vi "ExtTrigAuger.vi"() -> ()   [LabVIEW 2014]
uses:
  FPGA state.ctl
  <vilib>/Platform/TimedLoop/XDataNode/timing_clust.ctl
  <vilib>/Platform/TimedLoop/XDataNode/nitl_modes.ctl
  <vilib>/Platform/TimedLoop/XDataNode/wakeup.ctl
  <vilib>/rvi/Emulation/niFpgaSctlEmulationGetInTimedLoop.vi
  <vilib>/rvi/Emulation/niFpgaEmulationReportErrorSimple.vi
  <vilib>/rvi/Emulation/niFpgaGetClockAttributes.vi
  <vilib>/rvi/Emulation/niFpgaCriticalErrorInLSC.vi
  <vilib>/rvi/eio/common/nirviEmuTemplateMethod_errors.vi
  <vilib>/rvi/interface/RandomDataEmulation/niFpgaRandomDataHandleErrors.vi
  <vilib>/Platform/TimedLoop/XDataNode/XDataNode.xnode
  <vilib>/eio/EIONode/EIONode.xnode
  <vilib>/rvi/DataTransferAndStorage/Container/XNode/niFpgaContainer.xnode
  <vilib>/rvi/interface/RandomDataEmulation/nirviRandomDataFpgaReadWriteTemplate.vi
  <vilib>/Platform/TimedLoop/XDataNode/XDNodeRunTimeDep.lvlib
panel:
  out "Overflow":bool
  in  "Trigger Mode":enum8{"Off", "PXI Trig0", "DIO-08 Trig"}(ring)
  # "Acquisition can be controlled by external trigger\n(through PXI backplane or input connector)\nor by the FPGA 25 MHz Clock."
  # "ExtTrig AugerCounter"
  # "Each U64 FIFO element is a pair of U32 with\n28 bits data, 4 bit ID in most significant bits\nID 0-7 for data channels, 8 for clock and 9 for trig count\n\nOn trigger return sample count, delta T in first element,\nand counts since last trigger on the eight data channels\n(7 for Auger plus aux) in the next 4 elements\n\nOn overflow, set trigger mode to off and flush FIFO\nOFF mode clears overflow, also resests sample count"
  # "Red for overflow\ngreen for normal"
  # "FPGA DMA-FIFO CANNOT be cleared by FPGA,\nonly by PC Host VI. Ctr Overflow will be on when\nFPGA-side FIFO is full!"
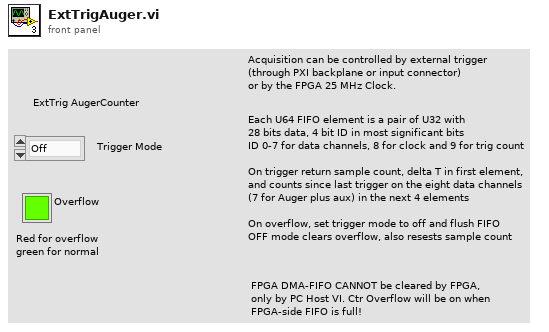
[diagram p1: front panel]
types:
  T1 = typedef "FPGA state.ctl" = enum8{"Wait", "Triggered", "Transfer 1", "Transfer 2", "Transfer 3", "Transfer 4", "Overflow"}
  T2 = typedef "XDNodeRunTimeDep.lvlib/timing_clust.ctl" = cluster{"Expected End [f-1]":u64, "Actual End [f-1]":u64, "Finished Late? [f-1]":bool, "Expected End [i-1]":u64, "Actual End [i-1]":u64, "Finished Late? [i-1]":bool, "Expected Start [i]":u64, "Actual Start [i]":u64, "Expected Start [f]":u64, "Actual Start [f]":u64, "Source Name":string, "Structure Name":string, "Period":i64, "Deadline":i64, "Offset":i64, "Start":i64, "Priority":i32, "Timeout":i32, "Mode":T3, "Wakeup Reason":T4, "Error":errorcluster, "Source Type":string, "Secondary Source Type":string, "Global End Time":u64, "Global Start Time":u64, "Frame Duration":u64, "Iteration Duration":u64, "Assigned CPU":i32, "I/O Scan Engine Mode":u32}
  T3 = typedef "XDNodeRunTimeDep.lvlib/nitl_modes.ctl" = enum32{"No Change", "Process missed periods, maintain original phase", "Discard missed periods, maintain original phase", "Process missed periods, ignore original phase", "Discard missed periods, ignore original phase"}
  T4 = typedef "XDNodeRunTimeDep.lvlib/wakeup.ctl" = enum32{"Normal", "Aborted", "Asynchronous wakeup", "Timing source error", "Timed loop error", "Timeout"}
  T5 = enum16{"Off", "PXI Trig0", "DIO-08 Trig", "Clocked"}
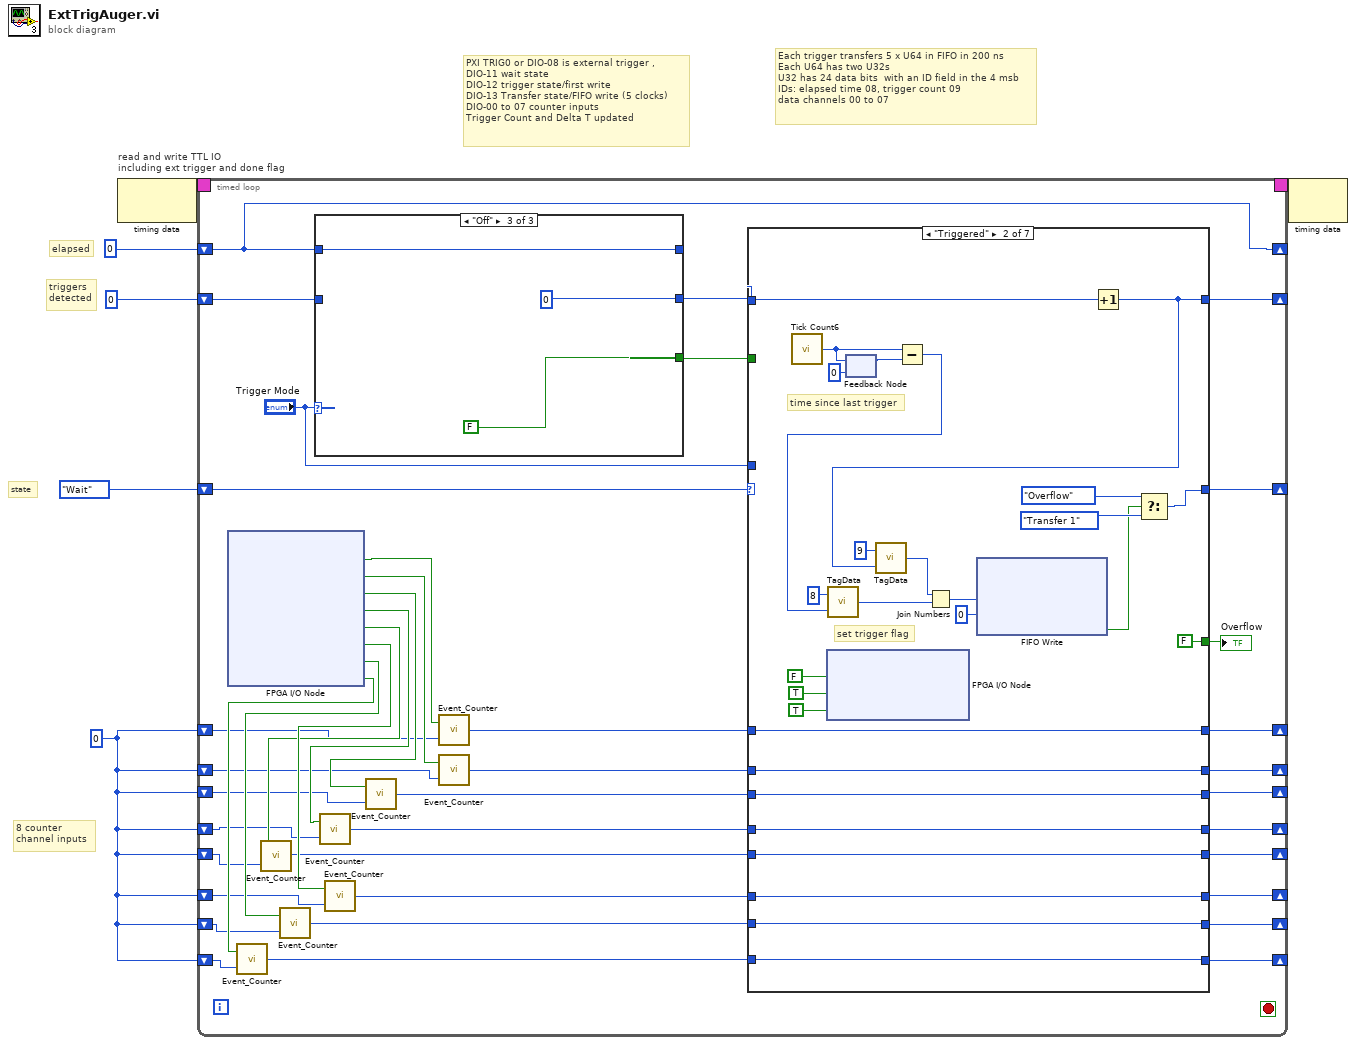
[diagram p0: block diagram]
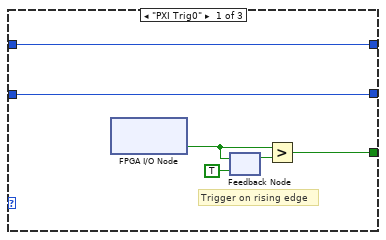
[diagram p2: hidden frame]
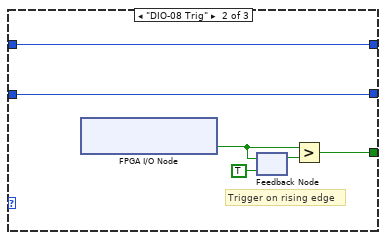
[diagram p3: hidden frame]
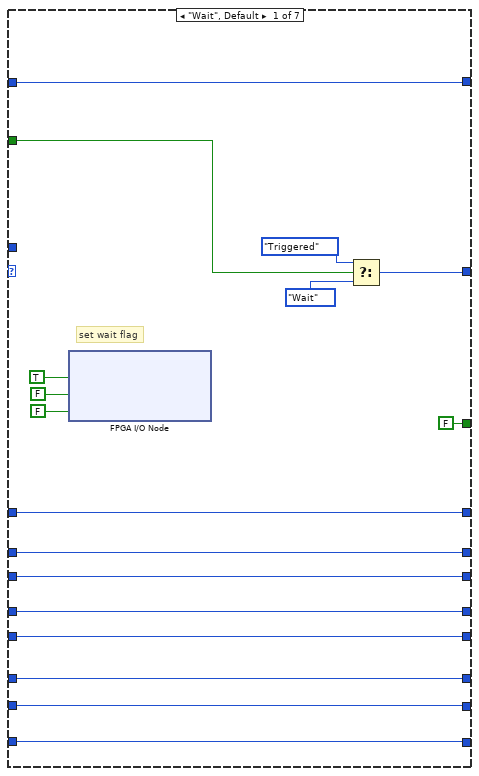
[diagram p4: hidden frame]
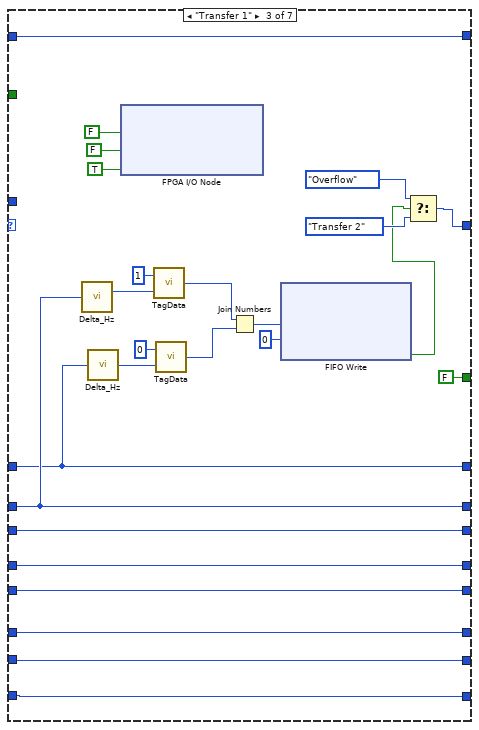
[diagram p5: hidden frame]
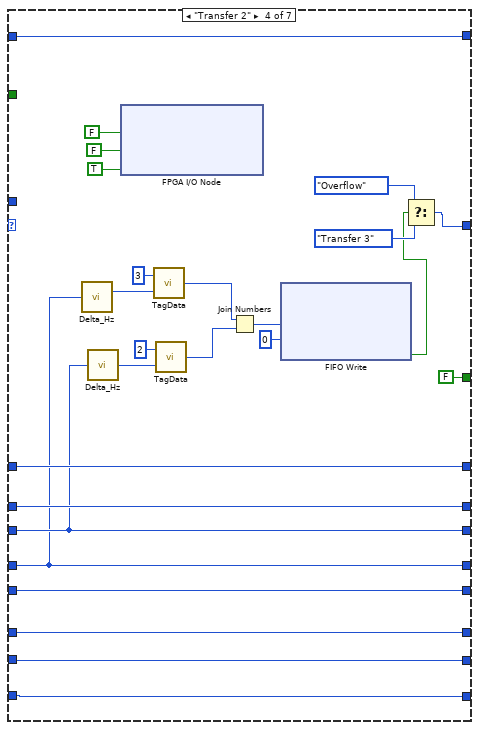
[diagram p6: hidden frame]
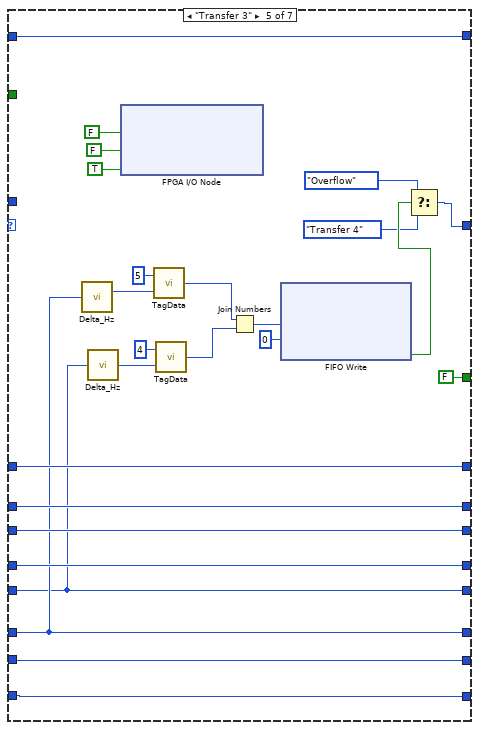
[diagram p7: hidden frame]
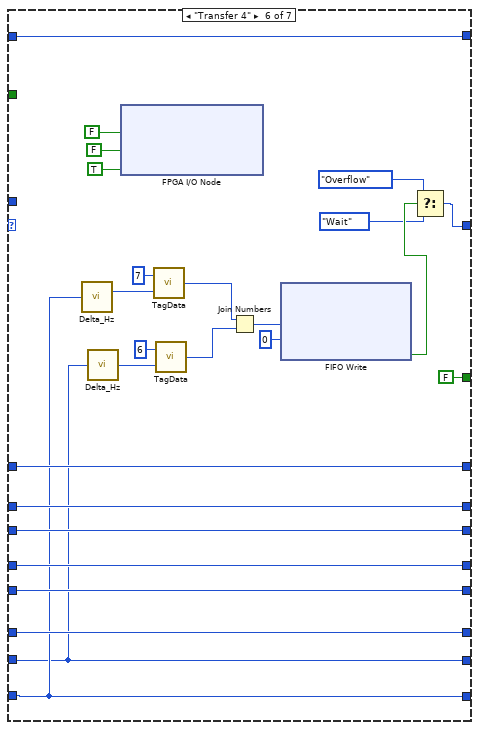
[diagram p8: hidden frame]
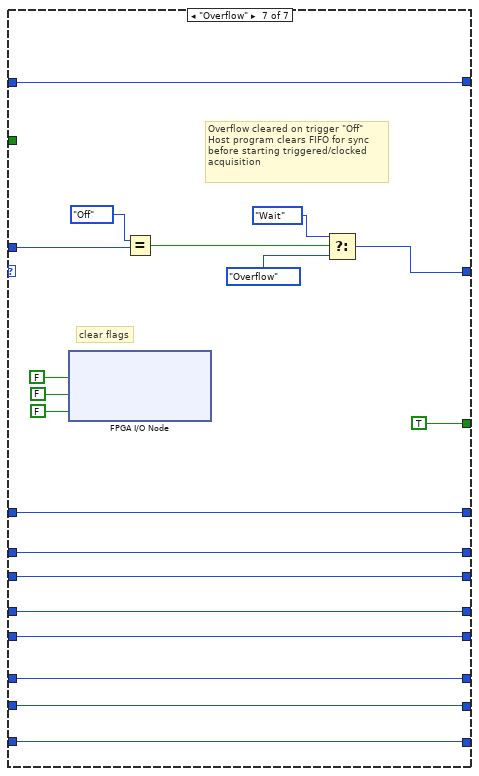
[diagram p9: hidden frame]
diagram:
  w1 = u32 0 ("Counts out")
  # "Each trigger transfers 5 x U64 in FIFO in 200 ns\nEach U64 has two U32s\nU32 has 24 data bits  with an ID field in the 4 msb\nIDs: elapsed time 08, trigger count 09\ndata channels 00 to 07"
  # "8 counter\nchannel inputs"
  # "elapsed"
  # "state"
  # "triggers\ndetected"
  # "PXI TRIG0 or DIO-08 is external trigger ,\nDIO-11 wait state\nDIO-12 trigger state/first write \nDIO-13 Transfer state/FIFO write (5 clocks)\nDIO-00 to 07 counter inputs \nTrigger Count and Delta T updated"
  n1 = node-c288() -> (w6:T2)  [unwired: 1 in]
  n2 = timed-loop "read and write TTL IO\nincluding ext trigger and done flag" {
    timing: w6 -> [_]
    timing-out: [_] -> w5
    shift-right: [w46] -> _
    shift-left: FPGA_state."Wait" -> [w47]
    shift-right: [w45] -> _
    shift-left: u32 0 -> [w11]
    shift-right: [w7] -> _
    shift-left: u32 0 -> [w7]
    shift-right: [w13] -> _
    shift-left: w1 -> [w29]
    shift-right: [w16] -> _
    shift-left: w1 -> [w30]
    shift-right: [w15] -> _
    shift-left: w1 -> [w34]
    shift-right: [w19] -> _
    shift-left: w1 -> [w35]
    shift-right: [w22] -> _
    shift-left: w1 -> [w38]
    shift-right: [w23] -> _
    shift-left: w1 -> [w37]
    shift-right: [w26] -> _
    shift-left: w1 -> [w39]
    shift-right: [w27] -> _
    shift-left: w1 -> [w40]
    stop <- _ stop-if-true
    n3 = xnode "FPGA I/O Node"() -> ("Connector0/DIO0"=w31:bool, "Connector0/DIO1"=w32:bool, "Connector0/DIO2"=w33:bool, "Connector0/DIO3"=w36:bool, "Connector0/DIO4"=w41:bool, "Connector0/DIO5"=w42:bool, "Connector0/DIO6"=w43:bool, "Connector0/DIO7"=w44:bool)  [unwired: 8 in, 8 out]
    n4 = call "Event_Counter.vi"("Counts in"=w40, "input"=w44) -> ("Counts out"=w28:u32)
    n5 = call "Event_Counter.vi"("Counts in"=w38, "input"=w41) -> ("Counts out"=w21:u32)
    n6 = call "Event_Counter.vi"("Counts in"=w39, "input"=w43) -> ("Counts out"=w25:u32)
    n7 = case shown="\"Off\"" "Trigger Mode" {
      tunnel: [w49 w56 FALSE ("Connector0/DIO8")] -> w8
      tunnel: w11 -> [w53 w59 _]
      tunnel: [w53 w59 u32 0] -> w9
      tunnel: w7 -> [w48 w54 w60]
      tunnel: [w48 w54 w60] -> _
      frame "PXI Trig0" {
        # "Trigger on rising edge"
        n8 = xnode "FPGA I/O Node"() -> ("TRIG0"=w50:bool)  [unwired: 1 in, 1 out]
        n9 = feedback #1(TRUE ("set")) -> (w51:bool)
        n10 = feedback-in #1(w50) -> ()
        n11 = Greater?(x=w50, y=w51) -> (0:w49:bool)
      }
      frame "DIO-08 Trig" {
        # "Trigger on rising edge"
        n12 = xnode "FPGA I/O Node"() -> ("Connector0/DIO8"=w55:bool)  [unwired: 1 in, 1 out]
        n13 = feedback #2(TRUE ("set")) -> (w58:bool)
        n14 = feedback-in #2(w55) -> ()
        n15 = Greater?(x=w55, y=w58) -> (0:w56:bool)
      }
      frame "Off" {
      }
    }
    n16 = call "Event_Counter.vi"("Counts in"=w35, "input"=w36) -> ("Counts out"=w20:u32)
    n17 = call "Event_Counter.vi"("Counts in"=w37, "input"=w42) -> ("Counts out"=w24:u32)
    n18 = call "Event_Counter.vi"("Counts in"=w34, "input"=w33) -> ("Counts out"=w18:u32)
    n19 = call "Event_Counter.vi"("Counts in"=w29, "input"=w31) -> ("Counts out"=w14:u32)
    n20 = call "Event_Counter.vi"("Counts in"=w30, "input"=w32) -> ("Counts out"=w17:u32)
    n21 = case shown="\"Triggered\"" w47 {
      tunnel: [w77 w85 w109 w134 w159 w184 w208] -> w46
      tunnel: w9 -> [w75 w107 w125 w150 w175 w200 w226]
      tunnel: [w75 w86 w125 w150 w175 w200 w226] -> w45
      tunnel: w8 -> [w76 _ _ _ _ _ _]
      tunnel: w28 -> [w74 w100 w118 w144 w171 w189 w225]
      tunnel: [w74 w100 w118 w144 w171 w189 w225] -> w27
      tunnel: [w73 w99 w119 w145 w172 w188 w224] -> w26
      tunnel: w25 -> [w73 w99 w119 w145 w172 w188 w224]
      tunnel: w24 -> [w72 w98 w120 w146 w164 w191 w223]
      tunnel: [w72 w98 w120 w146 w164 w191 w223] -> w23
      tunnel: [w71 w97 w121 w147 w163 w190 w222] -> w22
      tunnel: w21 -> [w71 w97 w121 w147 w163 w190 w222]
      tunnel: w20 -> [w70 w93 w117 w138 w165 w192 w221]
      tunnel: [w70 w93 w117 w138 w165 w192 w221] -> w19
      tunnel: w18 -> [w68 w96 w122 w139 w166 w193 w219]
      tunnel: w17 -> [w69 w95 w114 w141 w168 w195 w220]
      tunnel: [w69 w95 w114 w141 w168 w195 w220] -> w16
      tunnel: [w68 w96 w122 w139 w166 w193 w219] -> w15
      tunnel: w14 -> [w67 w94 w113 w140 w167 w194 w218]
      tunnel: [w67 w94 w113 w140 w167 w194 w218] -> w13
      tunnel: [FALSE ("Connector0/DIO11") FALSE ("Connector0/DIO11") FALSE ("Connector0/DIO11") FALSE ("Connector0/DIO11") FALSE ("Connector0/DIO11") FALSE ("Connector0/DIO11") TRUE ("Connector0/DIO11")] -> w12
      tunnel: "Trigger Mode" -> [_ _ _ _ _ _ w213]
      frame "Wait", Default {
        # "set wait flag"
        n22 = xnode "FPGA I/O Node"("Connector0/DIO11"=TRUE, "Connector0/DIO12"=FALSE ("Connector0/DIO11"), "Connector0/DIO13"=FALSE ("Connector0/DIO11")) -> ()  [unwired: 3 in, 3 out]
        n23 = Select(t=FPGA_state."Triggered", s=w76, f=FPGA_state."Wait") -> (s? t:f=w77:T1)
      }
      frame "Triggered" {
        # "time since last trigger"
        # "set trigger flag"
        n24 = Increment(x=w107) -> ()  [unwired: 1 out]
        n25 = call "Tick Count6"() -> ("Tick Count(Ticks)"=w105:u32)
        n26 = xnode "FPGA I/O Node"("Connector0/DIO11"=FALSE, "Connector0/DIO12"=TRUE ("Connector0/DIO11"), "Connector0/DIO13"=TRUE ("Connector0/DIO11")) -> ()  [unwired: 3 in, 3 out]
        n27 = feedback-in #3(w105) -> ()
        n28 = feedback #3(u32 0 ("Tick Count(Ticks)")) -> (w106:u32)
        n29 = Subtract(x=w105, y=w106) -> (x-y=w80:u32)
        n30 = call "TagData.vi"("Data"=w80, "Tag"=u8 8) -> ("Data 2"=w87:u32)
        n31 = Increment(x=w107) -> (x+1=w86:u32)
        n32 = call "TagData.vi"("Data"=w86, "Tag"=u8 9) -> ("Data 2"=w90:u32)
        n33 = Join Numbers(hi=w90, lo=w87) -> ((hi.lo)=w92:u64)
        n34 = xnode ("FIFO Write")("Element"=w92, "Timeout"=0) -> ("Timed Out?"=w82:bool)  [unwired: 1 in, 1 out]
        n35 = Select(t=FPGA_state."Overflow", s=w82, f=FPGA_state."Transfer 1") -> (s? t:f=w85:T1)
      }
      frame "Transfer 1" {
        n36 = call "Delta_Hz.vi"("Counts"=w114) -> ("Delta"=w115:u32)
        n37 = call "Delta_Hz.vi"("Counts"=w113) -> ("Delta"=w116:u32)
        n38 = xnode "FPGA I/O Node"("Connector0/DIO11"=FALSE ("Connector0/DIO15"), "Connector0/DIO12"=FALSE ("Connector0/DIO15"), "Connector0/DIO13"=TRUE ("Connector0/DIO15")) -> ()  [unwired: 3 in, 3 out]
        n39 = call "TagData.vi"("Data"=w115, "Tag"=u8 1) -> ("Data 2"=w127:u32)
        n40 = call "TagData.vi"("Data"=w116, "Tag"=u8 0) -> ("Data 2"=w123:u32)
        n41 = Join Numbers(hi=w127, lo=w123) -> ((hi.lo)=w132:u64)
        n42 = xnode ("FIFO Write")("Element"=w132, "Timeout"=0) -> ("Timed Out?"=w110:bool)  [unwired: 1 in, 1 out]
        n43 = Select(t=FPGA_state."Overflow", s=w110, f=FPGA_state."Transfer 2") -> (s? t:f=w109:T1)
      }
      frame "Transfer 2" {
        n44 = call "Delta_Hz.vi"("Counts"=w138) -> ("Delta"=w142:u32)
        n45 = call "Delta_Hz.vi"("Counts"=w139) -> ("Delta"=w143:u32)
        n46 = xnode "FPGA I/O Node"("Connector0/DIO11"=FALSE ("Connector0/DIO15"), "Connector0/DIO12"=FALSE ("Connector0/DIO15"), "Connector0/DIO13"=TRUE ("Connector0/DIO15")) -> ()  [unwired: 3 in, 3 out]
        n47 = call "TagData.vi"("Data"=w142, "Tag"=u8 3) -> ("Data 2"=w152:u32)
        n48 = call "TagData.vi"("Data"=w143, "Tag"=u8 2) -> ("Data 2"=w148:u32)
        n49 = Join Numbers(hi=w152, lo=w148) -> ((hi.lo)=w157:u64)
        n50 = xnode ("FIFO Write")("Element"=w157, "Timeout"=0) -> ("Timed Out?"=w136:bool)  [unwired: 1 in, 1 out]
        n51 = Select(t=FPGA_state."Overflow", s=w136, f=FPGA_state."Transfer 3") -> (s? t:f=w134:T1)
      }
      frame "Transfer 3" {
        n52 = call "Delta_Hz.vi"("Counts"=w164) -> ("Delta"=w169:u32)
        n53 = call "Delta_Hz.vi"("Counts"=w163) -> ("Delta"=w170:u32)
        n54 = xnode "FPGA I/O Node"("Connector0/DIO11"=FALSE ("Connector0/DIO15"), "Connector0/DIO12"=FALSE ("Connector0/DIO15"), "Connector0/DIO13"=TRUE ("Connector0/DIO15")) -> ()  [unwired: 3 in, 3 out]
        n55 = call "TagData.vi"("Data"=w169, "Tag"=u8 5) -> ("Data 2"=w177:u32)
        n56 = call "TagData.vi"("Data"=w170, "Tag"=u8 4) -> ("Data 2"=w173:u32)
        n57 = Join Numbers(hi=w177, lo=w173) -> ((hi.lo)=w182:u64)
        n58 = xnode ("FIFO Write")("Element"=w182, "Timeout"=0) -> ("Timed Out?"=w162:bool)  [unwired: 1 in, 1 out]
        n59 = Select(t=FPGA_state."Overflow", s=w162, f=FPGA_state."Transfer 4") -> (s? t:f=w159:T1)
      }
      frame "Transfer 4" {
        n60 = call "Delta_Hz.vi"("Counts"=w189) -> ("Delta"=w196:u32)
        n61 = call "Delta_Hz.vi"("Counts"=w188) -> ("Delta"=w197:u32)
        n62 = xnode "FPGA I/O Node"("Connector0/DIO11"=FALSE ("Connector0/DIO15"), "Connector0/DIO12"=FALSE ("Connector0/DIO15"), "Connector0/DIO13"=TRUE ("Connector0/DIO15")) -> ()  [unwired: 3 in, 3 out]
        n63 = call "TagData.vi"("Data"=w196, "Tag"=u8 7) -> ("Data 2"=w202:u32)
        n64 = call "TagData.vi"("Data"=w197, "Tag"=u8 6) -> ("Data 2"=w198:u32)
        n65 = Join Numbers(hi=w202, lo=w198) -> ((hi.lo)=w207:u64)
        n66 = xnode ("FIFO Write")("Element"=w207, "Timeout"=0) -> ("Timed Out?"=w187:bool)  [unwired: 1 in, 1 out]
        n67 = Select(t=FPGA_state."Overflow", s=w187, f=FPGA_state."Wait") -> (s? t:f=w184:T1)
      }
      frame "Overflow" {
        # "Overflow cleared on trigger \"Off\"\nHost program clears FIFO for sync\nbefore starting triggered/clocked\nacquisition"
        # "clear flags"
        n68 = xnode "FPGA I/O Node"("Connector0/DIO11"=FALSE, "Connector0/DIO12"=FALSE ("Connector0/DIO11"), "Connector0/DIO13"=FALSE ("Connector0/DIO11")) -> ()  [unwired: 3 in, 3 out]
        n69 = Equal?(x=T5."Off" ("Trigger Mode"), y=w213) -> (x = y?=w211:bool)
        n70 = Select(t=FPGA_state."Wait", s=w211, f=FPGA_state."Overflow") -> (s? t:f=w208:T1)
      }
    }
    "Overflow" <- w12
  }
  n71 = node-c288(w5) -> ()  [unwired: 1 out]
